vi "MAVLink Recieved Param.vi"(7 "FGV Method":T2, 11 "Param Value":T1) -> (3 "Param Value Out":T1)   [LabVIEW 2014]
uses:
  Controls/FGV Methods.ctl
  MAVLink/Controls/MAVLink Recieved Param.ctl
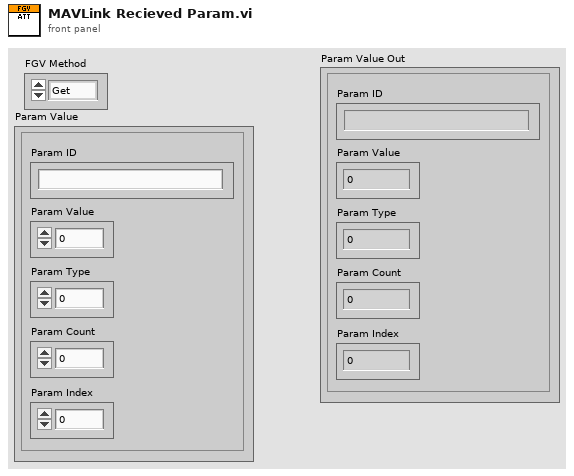
[diagram p1: front panel]
types:
  T1 = typedef "MAVLink Recieved Param.ctl" = cluster{"Param ID":string, "Param Value":sgl, "Param Type":u8, "Param Count":u16, "Param Index":u16}
  T2 = typedef "FGV Methods.ctl" = enum16{"Get", "Set"}
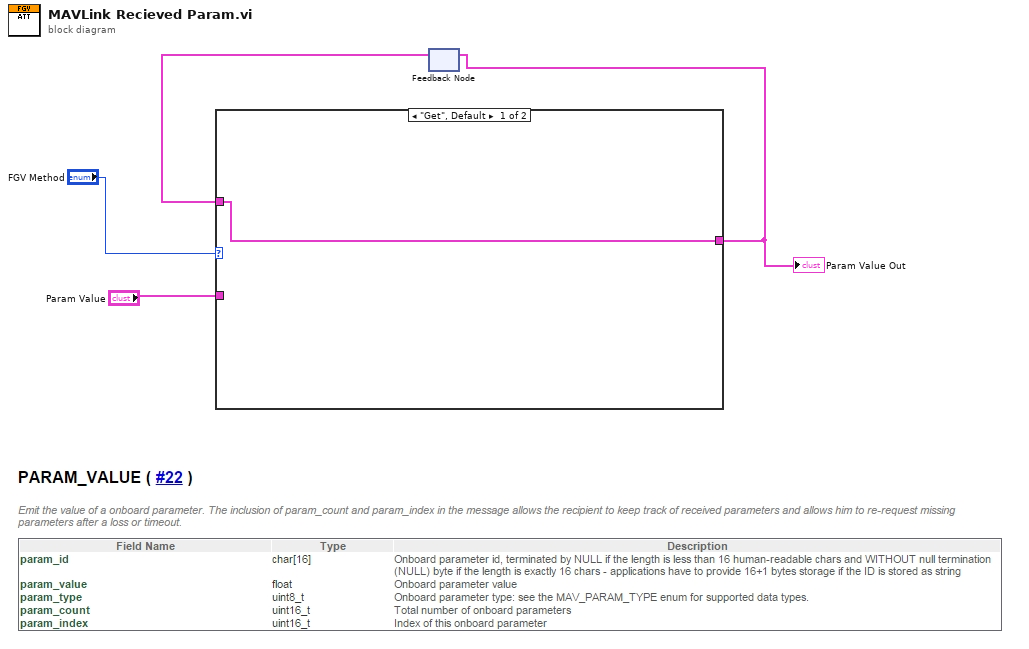
[diagram p0: block diagram]
diagram:
  n1 = feedback #1() -> (w2:T1)  [unwired: 1 in]
  n2 = case shown="\"Get\", Default" "FGV Method" {
    tunnel: "Param Value" -> [_ w6]
    tunnel: [w5 w6] -> w3
    tunnel: w2 -> [w5 _]
    frame "Get", Default {
    }
    frame "Set" {
    }
  }
  "Param Value Out" <- w3
  n3 = feedback-in #1(w3) -> ()
